vi "Export Result Table to CSV.vi"(6 "IsCalibration":bool, 7 "Limit Status":T1, 8 "error in":errorcluster, 9 "Data String":string[][](array[string]), 10 "Col Header String":string[](array[string]), 11 "GU Pass Count Indicator":refnum<vi>) -> (0 "error out":errorcluster, 1 "Data String dup":string[][](array[string]), 2 "Col Header String dup":string[](array[string]))   [LabVIEW 2020, in "GUCalibration2.lvlib"]
doc: "Export GU Pass Count (as first two comment lines) and Result Table (as csv table) to CSV file. A column of Cal Limit Failed or Check Limit Failed will be added into the table.."
uses:
  GUCalibration2.lvlib
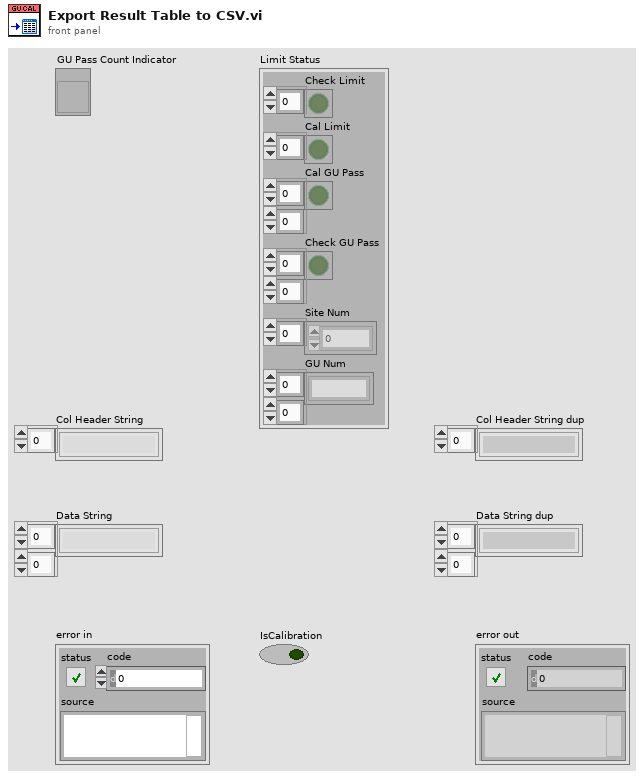
[diagram p1: front panel]
types:
  T1 = cluster{"Check Limit":bool[], "Cal Limit":bool[], "Cal GU Pass":bool[][], "Check GU Pass":bool[][], "Site Num":i32[], "GU Num":string[][]}
  T2 = enum16{"open", "replace", "create", "open or create", "replace or create", "replace or create with confirmation"}
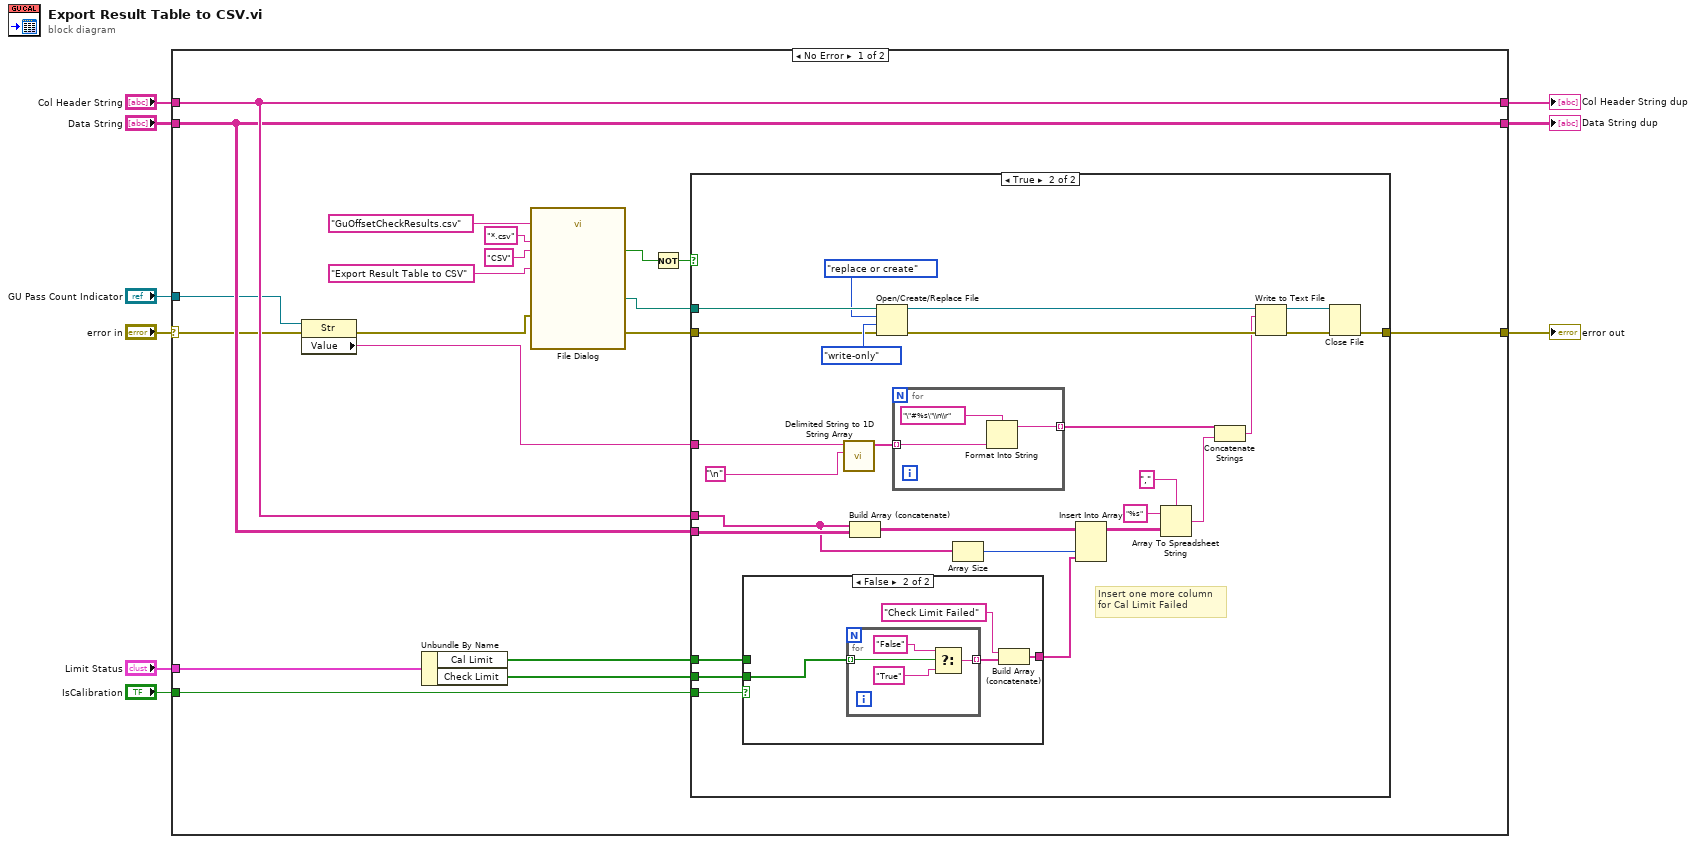
[diagram p0: block diagram]
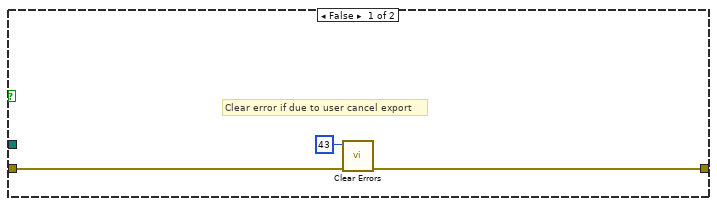
[diagram p2: hidden frame]
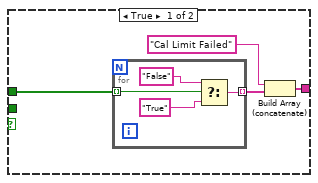
[diagram p3: hidden frame]
diagram:
  n1 = case shown="No Error" "error in" {
    selector: "error in" -> [w19 w79]
    tunnel: "Col Header String" -> [w21 w78]
    tunnel: "Data String" -> [w20 w77]
    tunnel: [w15 w79] -> w7
    tunnel: [w21 w78] -> w6
    tunnel: [w20 w77] -> w5
    tunnel: "GU Pass Count Indicator" -> [w18 _]
    tunnel: "Limit Status" -> [w13 _]
    tunnel: "IsCalibration" -> [w12 _]
    frame No Error {
      n2 = property class="Str"(reference=w18, error in=w19) -> (error out=w17:errorcluster, "Value"=w16:string)  [unwired: 1 out]
      n3 = Unbundle By Name(w13) -> ("Cal Limit"=w11:bool[], "Check Limit"=w10:bool[])
      n4 = call "File Dialog"("prompt"="Export Result Table to CSV", "default name"="GuOffsetCheckResults.csv", "error in"=w17, "pattern (all files)"="*.csv", "pattern label"="CSV") -> ("selected path"=w22:path, "cancelled"=w24:bool, "error out"=w14:errorcluster)  [unwired: 7 in, 1 out]
      n5 = Not(x=w24) -> (.not. x?=w23:bool)
      n6 = case shown="True" w23 {
        tunnel: w22 -> [_ w57]
        tunnel: w21 -> [_ w36]
        tunnel: w20 -> [_ w54]
        tunnel: w16 -> [_ w53]
        tunnel: [w30 w43] -> w15
        tunnel: w14 -> [w31 w42]
        tunnel: w12 -> [_ w40]
        tunnel: w11 -> [_ w39]
        tunnel: w10 -> [_ w33]
        frame False {
          # "Clear error if due to user cancel export"
          n7 = call <vilib>:"Clear Errors.vi"("error in (no error)"=w31, "specific error code to clear (0: all)"=43) -> ("error out"=w30:errorcluster)  [unwired: 4 in, 1 out]
        }
        frame True {
          # "Insert one more column\nfor Cal Limit Failed"
          n8 = case shown="False" w40 {
            tunnel: w39 -> [w61 _]
            tunnel: [w58 w67] -> w34
            tunnel: w33 -> [_ w66]
            frame True {
              n9 = for {
                tunnel: w61 -> [w63] mode=indexing
                tunnel: [w62] -> w60 mode=indexing
                n10 = Select(t="False", s=w63, f="True") -> (s? t:f=w62:string)
              }
              n11 = Build Array (concatenate)("Cal Limit Failed", w60) -> (w58:string[])
            }
            frame False {
              n12 = for {
                tunnel: w66 -> [w71] mode=indexing
                tunnel: [w70] -> w69 mode=indexing
                n13 = Select(t="False", s=w71, f="True") -> (s? t:f=w70:string)
              }
              n14 = Build Array (concatenate)("Check Limit Failed", w69) -> (w67:string[])
            }
          }
          n15 = call <vilib>:"Delimited String to 1D String Array.vi"("delimiter"="\n", "delimited string"=w53) -> ("string array"=w50:string[])  [unwired: 9 in]
          n16 = Build Array (concatenate)(w36, w54) -> (w37:string[][])
          n17 = Open/Create/Replace File(file path (use dialog)=w57, error in=w42, operation (0:open)=T2."replace or create", access (0:read/write)=enum16{"read/write", "read-only", "write-only"}."write-only") -> (refnum out=w47:refnum<file>, error out=w46:errorcluster)  [unwired: 2 in, 1 out]
          n18 = for {
            tunnel: w50 -> [w76] mode=indexing
            tunnel: [w74] -> w49 mode=indexing
            n19 = Format Into String(format string="\"#%s\"\\n\\r", w76) -> (resulting string=w74:string)  [unwired: 2 in, 1 out]
          }
          n20 = Array Size(array=w36) -> (size(s)=w35:i32)
          n21 = Insert Into Array(array=w37, index (col)=w35, new element=w34) -> (w38:string[][])  [unwired: 1 in]
          n22 = Array To Spreadsheet String(delimiter (Tab)=",", array=w38, 3:"%s" ("format string")) -> (spreadsheet string=w48:string)
          n23 = Concatenate Strings(w49, w48) -> (w41:string)
          n24 = Write to Text File(file (use dialog)=w47, text=w41, error in=w46) -> (refnum out=w45:refnum<file>, error out=w44:errorcluster)  [unwired: 1 in, 1 out]
          n25 = Close File(refnum=w45, error in=w44) -> (error out=w43:errorcluster)  [unwired: 1 out]
        }
      }
    }
    frame Error {
    }
  }
  "error out" <- w7
  "Col Header String dup" <- w6
  "Data String dup" <- w5
